vi "Test.vi"() -> ()   [LabVIEW 2019, in "TEMPerHUM.lvlib"]
uses:
  TEMPerHUM.lvlib
  RDingUSB.dll
panel:
  out "Hum Chart":dbl(graph)
  out "DeviceHandle":i64(graph)
  out "Temp Chart":dbl(graph)
  out "error out":errorcluster
  out "Humidity":dbl
  out "Temperature":dbl
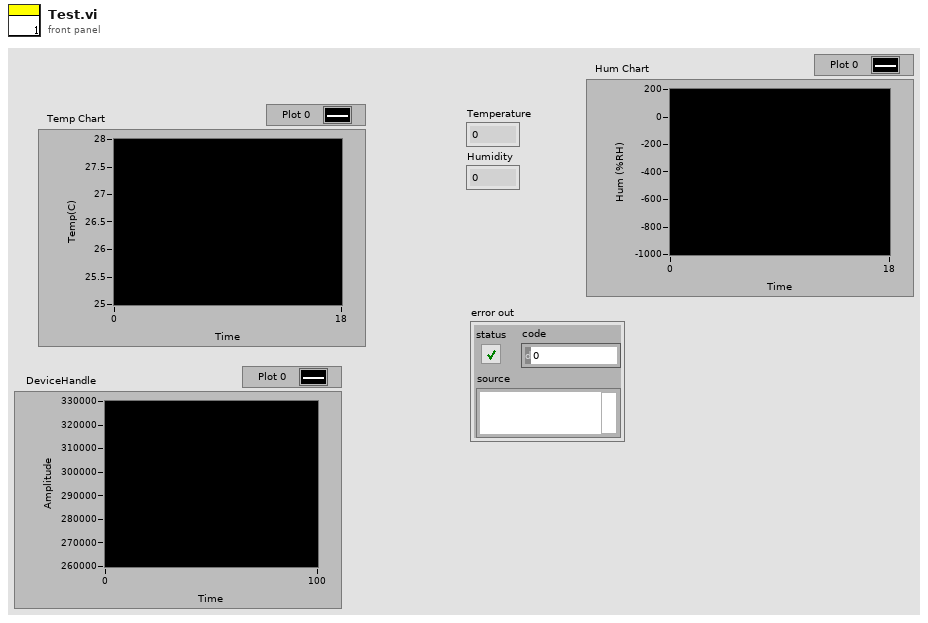
[diagram p1: front panel]
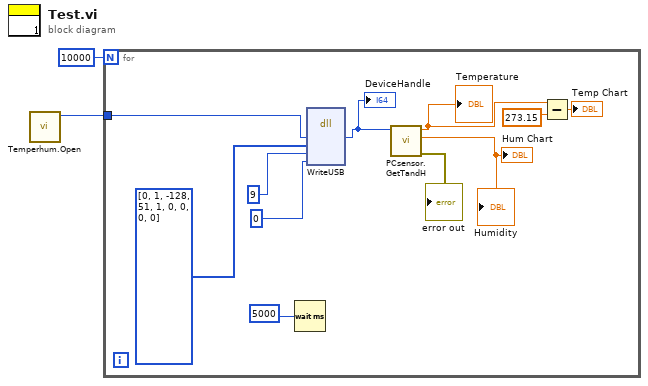
[diagram p0: block diagram]
diagram:
  n1 = call "Temperhum.Open.vi"() -> ("Device Handle"=w2:i64)  [unwired: 9 in, 2 out]
  n2 = for {
    N: 10000 -> [_]
    tunnel: w2 -> [w10]
    n3 = Wait (ms)(milliseconds to wait=u32 5000 ("millisecond timer value")) -> ()  [unwired: 1 out]
    n4 = dll-call lib="C:/Users/Ranjani/Documents/GitHub/Temperhum-Instrument/lvsrc/SMOs/TEMPerHUM/RDingUSB.dll" fn="WriteUSB"("deviceHandle"=w10, "buffer"=i8[] [0, 1, -128, 51, 1, 0, 0, 0, 0] ("Array"), "bytesCount"=9, "number0fBytesWrite"=u64 0) -> ("deviceHandle"=w7:i64)  [unwired: 7 in, 2 out]
    "DeviceHandle" <- w7
    n5 = call "PCsensor.GetTandH.vi"("Device Handle"=w7) -> ("error out"=→"error out":errorcluster, "Humidity"=→"Humidity" →"Hum Chart":dbl, "Temperature"=w4:dbl)  [unwired: 8 in]
    "Temperature" <- w4
    n6 = Subtract(x=w4, y=273.15 ("x")) -> (x-y=→"Temp Chart":dbl)
  }
